vi "Get Last Record (SubVI).vi"(3 "error in":errorcluster) -> (0 "error out":errorcluster, 1 "experiment record":i32, 2 "shot record":i32)   [LabVIEW 2015]
uses:
  <vilib>/addons/database/Connection.llb/DB Tools Open Connec (Path).vi
  <vilib>/addons/database/_DB Variant To Data/Database Variant To Data.xnode
  <vilib>/addons/database/NI_Database_API.lvlib
panel:
  out "App.Dir":path
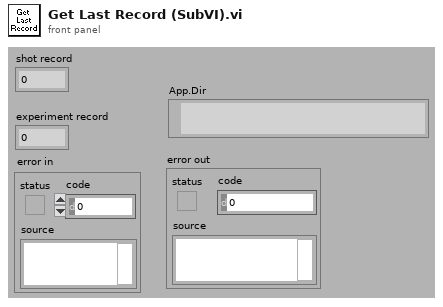
[diagram p1: front panel]
types:
  T1 = enum32{"invalid app kind", "Development System", "Run Time System", "Student Edition", "Embedded LabVIEW", "Evaluation", "Custom"}
  T2 = typedef "NI_Database_API.lvlib/Conn ObjectReference.ctl" = refnum<k1>
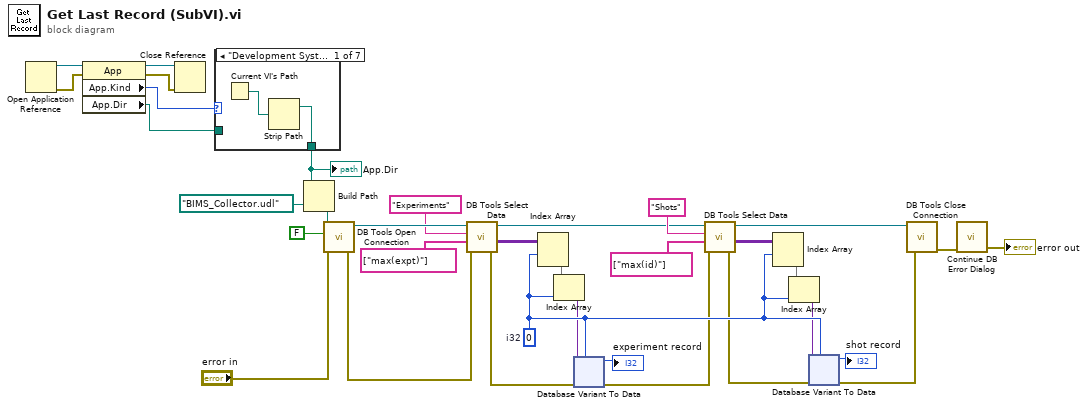
[diagram p0: block diagram]
diagram:
  w34 = 0  # i32
  n1 = Open Application Reference() -> (0:w5:errorcluster, 3:w6:refnum<vi>)  [unwired: 1 in, 3 out]
  n2 = property class="App"(reference=w6, error in=w5) -> (reference out=w4:refnum<vi>, error out=w3:errorcluster, "App.Kind"=w2:T1, "App.Dir"=w1:path)
  n3 = Close Reference(reference=w4, error in (no error)=w3) -> ()  [unwired: 1 out]
  n4 = case shown="\"Development System\"" w2 {
    tunnel: [w35 w37 w38 w39 w40 w41 w42] -> w7
    tunnel: w1 -> [_ w37 w38 w39 w40 w41 w42]
    frame "Development System" {
      n5 = Current VI's Path() -> (path=w36:path)
      n6 = Strip Path(path=w36) -> (stripped path=w35:path)  [unwired: 1 out]
    }
    frame "Run Time System" {
    }
    frame "Student Edition" {
    }
    frame "Embedded LabVIEW" {
    }
    frame "Evaluation" {
    }
    frame "Custom" {
    }
    frame "invalid app kind" {
    }
  }
  "App.Dir" <- w7
  n7 = Build Path(base path=w7, name or relative path=path "BIMS_Collector.udl" ("connectString")) -> (appended path=w9:path)
  n8 = call-poly <vilib>:"DB Tools Open Connection.vi"("error in (no error)"="error in", "prompt? (F)"=FALSE ("prompt? (f)"), "connection information"=w9) -> ("error out"=w29:errorcluster, "connection reference"=w31:T2)  [unwired: 2 in, 3 out]
  n9 = call <vilib>:"DB Tools Select Data.vi"("error in (no error)"=w29, "columns"=string[] ["max(expt)"], "table"="Experiments", "connection reference"=w31) -> ("error out"=w20:errorcluster, "data"=w14:variant[][], "connection reference out"=w16:T2)  [unwired: 2 out]
  n10 = Index Array(array=w14, index (row)=w34) -> (element=w13:variant[])  [unwired: 1 in]
  n11 = Index Array(array=w13, index=w34) -> (element=w15:variant)
  n12 = xnode "Database Variant To Data"("database variant"=w15, "error in"=w20, "type"=w34) -> ("data"=→"experiment record":i32, "error out"=w21:errorcluster)
  n13 = call <vilib>:"DB Tools Select Data.vi"("error in (no error)"=w21, "columns"=string[] ["max(id)"], "table"="Shots", "connection reference"=w16) -> ("error out"=w22:errorcluster, "data"=w24:variant[][], "connection reference out"=w17:T2)  [unwired: 2 out]
  n14 = Index Array(array=w24, index (row)=w34) -> (element=w25:variant[])  [unwired: 1 in]
  n15 = Index Array(array=w25, index=w34) -> (element=w26:variant)
  n16 = xnode "Database Variant To Data"("database variant"=w26, "error in"=w22, "type"=w34) -> ("data"=→"shot record":i32, "error out"=w23:errorcluster)
  n17 = call <vilib>:"DB Tools Close Connection.vi"("error in (no error)"=w23, "connection reference"=w17) -> ("error out"=w32:errorcluster)  [unwired: 5 out]
  n18 = call "Continue DB Error Dialog.vi"("error in (no error)"=w32) -> ("error out"=→"error out":errorcluster)  [unwired: 3 in, 2 out]
